vi "sine_source.vi"(2 "pause":bool, 3 "sine_control":T1) -> (0 "Terminate?":bool, 1 "output_signal / V":dbl)   [LabVIEW 2014]
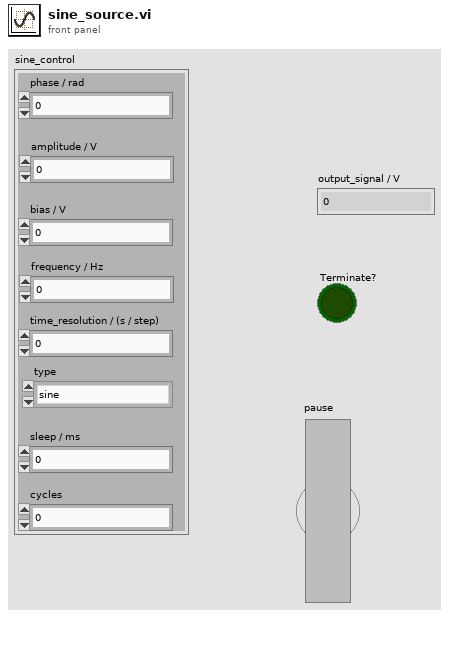
[diagram p1: front panel]
types:
  T1 = cluster{"amplitude / V":dbl, "frequency / Hz":dbl, "phase / rad":dbl, "type":enum16{"sine", "cosine", ""}, "sleep / ms":u32, "cycles":u32, "bias / V":dbl, "time_resolution / (s / step)":dbl}
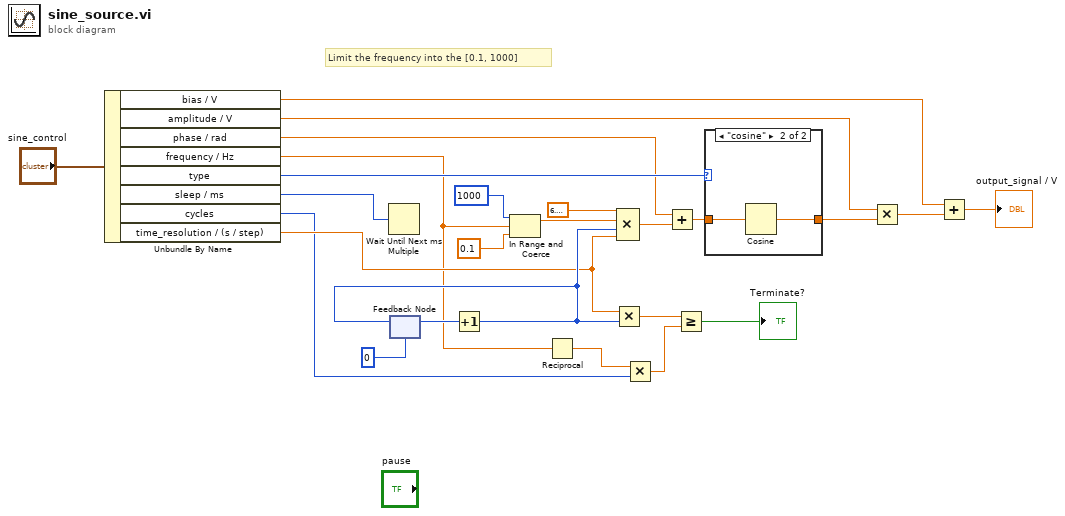
[diagram p0: block diagram]
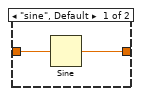
[diagram p2: hidden frame]
diagram:
  # "Limit the frequency into the [0.1, 1000]"
  n1 = Unbundle By Name("sine_control") -> ("bias / V"=w15:dbl, "amplitude / V"=w17:dbl, "phase / rad"=w20:dbl, "frequency / Hz"=w5:dbl, "type"=w24:enum16{"sine", "cosine", ""}, "sleep / ms"=w21:u32, "cycles"=w3:u32, "time_resolution / (s / step)"=w7:dbl)
  n2 = Wait Until Next ms Multiple(millisecond multiple=w21) -> ()  [unwired: 1 out]
  n3 = feedback #1(0) -> (w10:i32)
  n4 = Increment(x=w10) -> (x+1=w8:i32)
  n5 = feedback-in #1(w8) -> ()
  n6 = In Range and Coerce(upper limit=1000, x=w5, lower limit=0.1) -> (coerced(x)=w12:dbl)  [unwired: 1 out]
  n7 = Reciprocal(x=w5) -> (1/x=w4:dbl)
  n8 = Multiply(x=w7, y=w8) -> (x*y=w6:dbl)
  n9 = Compound Arithmetic op=MULTIPLY(6.283185307179586, w12, w8, w7) -> (w11:dbl)
  n10 = Multiply(x=w4, y=w3) -> (x*y=w2:dbl)
  n11 = Add(x=w20, y=w11) -> (x+y=w19:dbl)
  n12 = Greater Or Equal?(x=w6, y=w2) -> (x >= y?=→"Terminate?":bool)
  n13 = case shown="\"cosine\"" w24 {
    tunnel: w19 -> [w27 w29]
    tunnel: [w26 w28] -> w18
    frame "sine", Default {
      n14 = Sine(x=w27) -> (sin(x)=w26:dbl)
    }
    frame "cosine" {
      n15 = Cosine(x=w29) -> (cos(x)=w28:dbl)
    }
  }
  n16 = Multiply(x=w17, y=w18) -> (x*y=w16:dbl)
  n17 = Add(x=w15, y=w16) -> (x+y=→"output_signal / V":dbl)
